vi "Create Directory.vi"(6 "timeout (ms)":i32=30000, 8 "error in":errorcluster, 9 "create as needed":bool, 10 "remote path":string, 11 "session in":refnum<class "Session.lvclass">) -> (0 "error out":errorcluster, 3 "session out":refnum<class "Session.lvclass">)   [LabVIEW 2020, in "NI_SFTP.lvlib"]
doc: "Creates a remote directory."
uses:
  <vilib>/net/SFTP/NI_SFTP.lvlib
  <vilib>/net/SFTP/Session/Session.lvclass
  <vilib>/net/SFTP/API/Support/Command/SSH_FXP_MKDIR/Input.ctl
  <vilib>/net/SFTP/API/Support/File Attributes.ctl
  <vilib>/net/SFTP/File Attributes/File Attributes.lvclass/File Attributes.ctl
  <vilib>/net/SFTP/File Attributes/Read type.vi
  <vilib>/net/SFTP/File Attributes/Report item not found.vi
  <vilib>/Utility/error.llb/Error Cluster From Error Code.vi
  <vilib>/net/SFTP/File Attributes/File Attributes.lvclass
  <vilib>/Utility/Deadline/NI_Deadline.lvlib
  <vilib>/net/SFTP/API/Support/Command/SSH_FXP_MKDIR/SSH_FXP_MKDIR.lvclass
  <vilib>/net/SFTP/API/Support/Command/SSH_FXP_STAT/SSH_FXP_STAT.lvclass
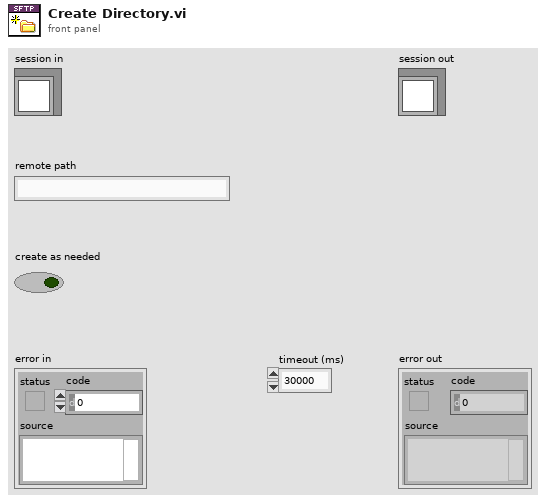
[diagram p1: front panel]
types:
  T1 = typedef "NI_SFTP.lvlib/SSH_FXP_MKDIR.lvclass/Input.ctl" = cluster{"path":string, "file attributes":T2}
  T2 = typedef "NI_SFTP.lvlib/File Attributes.ctl" = cluster{"SSH_FILEXFER_ATTR_SIZE":bool, "size":u64, "SSH_FILEXFER_ATTR_UIDGID":bool, "uid":u32, "gid":u32, "SSH_FILEXFER_ATTR_PERMISSIONS":bool, "permissions":u32, "SSH_FILEXFER_ATTR_ACMODTIME":bool, "atime":u32, "mtime":u32, "extended":map{string, string}}
  T3 = typedef "NI_Deadline.lvlib/Deadline.ctl" = cluster{"mode":T4, "deadline (ms)":u32}
  T4 = typedef "NI_Deadline.lvlib/Mode.ctl" = enum16{"Relative", "Use deadline", "Wait forever", "Nonblocking", "N/A"}
  T5 = typedef "NI_SFTP.lvlib/File Attributes.lvclass/File Type.ctl" = enum16{"File", "Directory", "Character device", "Block device", "Symbolic link", "Socket", "FIFO", "Unknown"}
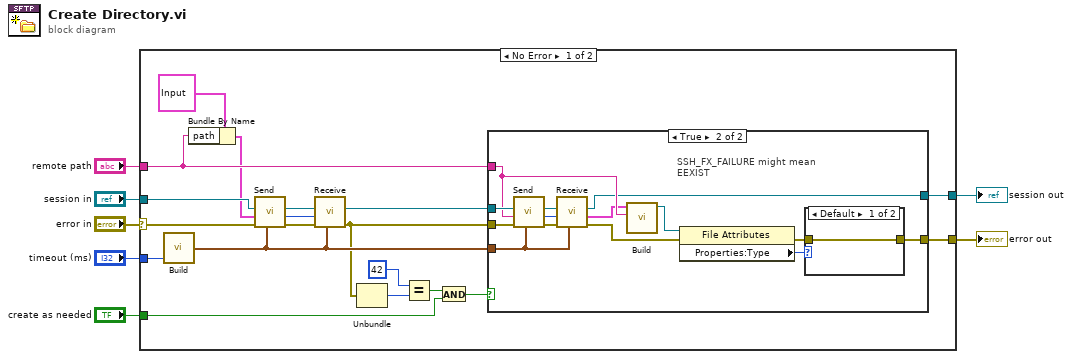
[diagram p0: block diagram]
diagram:
  n1 = case shown="No Error" "error in" {
    selector: "error in" -> [w24 w45]
    tunnel: [w21 w45] -> w6
    tunnel: [w22 w44] -> w4
    tunnel: "session in" -> [w13 w44]
    tunnel: "timeout (ms)" -> [w23 _]
    tunnel: "remote path" -> [w11 _]
    tunnel: "create as needed" -> [w19 _]
    frame No Error {
      n2 = call <vilib>:"Build.vi"("timeout (ms)"=w23) -> ("Deadline out"=w20:T3)  [unwired: 2 in]
      n3 = Bundle By Name(cluster=T1 {"path"="", "file attributes"={"SSH_FILEXFER_ATTR_SIZE"=FALSE, "size"=0, "SSH_FILEXFER_ATTR_UIDGID"=FALSE, "uid"=0, "gid"=0, "SSH_FILEXFER_ATTR_PERMISSIONS"=FALSE, "permissions"=0, "SSH_FILEXFER_ATTR_ACMODTIME"=FALSE, "atime"=0, "mtime"=0, "extended"={}}} ("input"), "path"=w11) -> (w10:T1)
      n4 = call <vilib>:"Send.vi"("deadline"=w20, "error in (no error)"=w24, "input"=w10, "session in"=w13) -> ("error out"=w25:errorcluster, "request id"=w9:u32, "session out"=w26:refnum<class "Session.lvclass">)  [unwired: 4 in, 1 out]
      n5 = call <vilib>:"Receive.vi"("Timeout"=w20, "error in (no error)"=w25, "request id"=w9, "session in"=w26) -> ("error out"=w17:errorcluster, "session out"=w8:refnum<class "Session.lvclass">)  [unwired: 4 in, 2 out]
      n6 = Unbundle(w17) -> ("code"=w15:i32)  [unwired: 2 out]
      n7 = Equal?(x=42, y=w15) -> (x = y?=w16:bool)
      n8 = And(x=w16, y=w19) -> (x .and. y?=w18:bool)
      n9 = case shown="True" w18 {
        tunnel: w8 -> [w28 w33]
        tunnel: [w28 w29] -> w22
        tunnel: [w27 w39] -> w21
        tunnel: w20 -> [_ w40]
        tunnel: w11 -> [_ w32]
        tunnel: w17 -> [w27 w38]
        frame False {
        }
        frame True {
          # "SSH_FX_FAILURE might mean EEXIST"
          n10 = call <vilib>:"Send.vi"("deadline"=w40, "error in (no error)"=w38, "path"=w32, "session in"=w33) -> ("error out"=w42:errorcluster, "request id"=w31:u32, "session out"=w41:refnum<class "Session.lvclass">)  [unwired: 4 in, 1 out]
          n11 = call <vilib>:"Receive.vi"("deadline"=w40, "error in (no error)"=w42, "request id"=w31, "session in"=w41) -> ("error out"=w36:errorcluster, "file attributes"=w30:T2, "session out"=w29:refnum<class "Session.lvclass">)  [unwired: 4 in, 1 out]
          n12 = call <vilib>:"Build.vi"("file name"=w32, "file attributes"=w30) -> ("file attributes out"=w37:refnum<class "File Attributes.lvclass">)  [unwired: 9 in]
          n13 = property class="File Attributes"(reference=w37, error in=w36) -> (error out=w35:errorcluster, "Properties:Type"=w34:T5)  [unwired: 1 out]
          n14 = case shown="Default" w34 {
            tunnel: w35 -> [w43 _]
            tunnel: [w43 _] -> w39
            frame Default {
            }
            frame "Directory" {
            }
          }
        }
      }
    }
    frame Error {
    }
  }
  "error out" <- w6
  "session out" <- w4
